vi "setEnabledState.vi"(0 "MultiAxisController in":refnum<class "_MultiAxisController.lvclass">, 1 "state (nc - for single-axis applications only)":bool, 2 "axes_states":T1, 5 "error in (no error)":errorcluster) -> (14 "MultiAxisController out":refnum<class "_MultiAxisController.lvclass">, 17 "success?":bool, 18 "response":string, 19 "error out":errorcluster)   [LabVIEW 2020, in "classes.lvlib" / "_MultiAxisController.lvclass"]
doc: "Produced By:\n\n<B>Kod Integrations, LLC</B>\n4835 Marianne Drive\nMount Airy, MD 21771\nhttp://www.kodintegrations.com\nemail: info@kodintegrations.com\nphone: (240) 687-1288"
uses:
  _MultiAxisController.lvclass
  C:/GEECS/Developers Version/source/Device Drivers/Newmark-NSC-A/Arcus Driver 3.0.0/ArcusUsbComm/classes/Controller/_Controller.lvclass
  motor_enabled_state_axes_group.ctl
  _Controller.lvclass
  common.lvlib
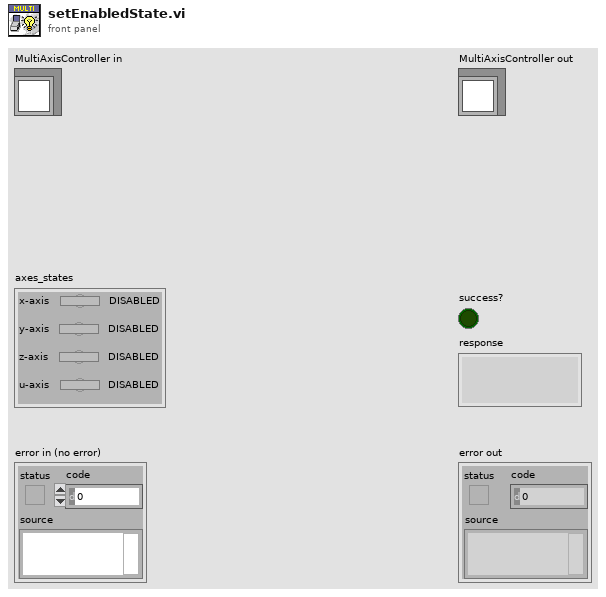
[diagram p1: front panel]
types:
  T1 = typedef "common.lvlib/motor_enabled_state_axes_group.ctl" = cluster{"x-axis":bool, "y-axis":bool, "z-axis":bool, "u-axis":bool}
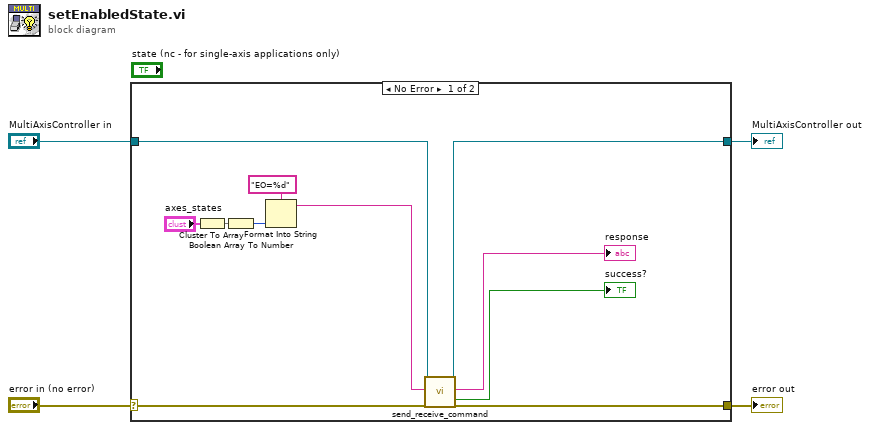
[diagram p0: block diagram]
diagram:
  n1 = case shown="No Error" "error in (no error)" {
    selector: "error in (no error)" -> [w11 w17]
    tunnel: [w10 w17] -> w3
    tunnel: [w8 w16] -> w1
    tunnel: "MultiAxisController in" -> [w9 w16]
    frame No Error {
      n2 = Cluster To Array(cluster="axes_states") -> (array=w14:bool[])
      n3 = Boolean Array To Number(Boolean array=w14) -> (number=w12:u32)
      n4 = Format Into String(format string="EO=%d", w12) -> (resulting string=w7:string)  [unwired: 2 in, 1 out]
      n5 = call "send_receive_command.vi"("reference (in)"=w9, "ASCII Command (in)"=w7, "error in (no error)"=w11) -> ("reference (out)"=w8:refnum<class "_MultiAxisController.lvclass">, "response (out)"=→"response":string, "success?"=→"success?":bool, "error out"=w10:errorcluster)  [unwired: 12 in, 1 out]
    }
    frame Error {
    }
  }
  "error out" <- w3
  "MultiAxisController out" <- w1
